vi "RTS Read System CFG.vi"(8 "Error In":errorcluster, 11 "Room CFG File Path":path) -> (0 "error out":errorcluster, 2 "Output Configuration":T1, 3 "Search File Path":path)   [LabVIEW 2020]
uses:
  Type Definitions/RTS Configuration Setup.ctl
  Type Definitions/RTS Wago Config.ctl
  Type Definitions/RTS APLUS Config.ctl
  Type Definitions/RTS Yokogawa MX Config.ctl
  Type Definitions/RTS Replay Server Control.ctl
  Type Definitions/RTS Server Configuration.ctl
  Type Definitions/RTS Station Settions TCP Comms.ctl
  Type Definitions/RTS Chamber Save Status.ctl
  Type Definitions/RTS Test Pattern.ctl
  <vilib>/Utility/file.llb/Read Delimited Spreadsheet (string).vi
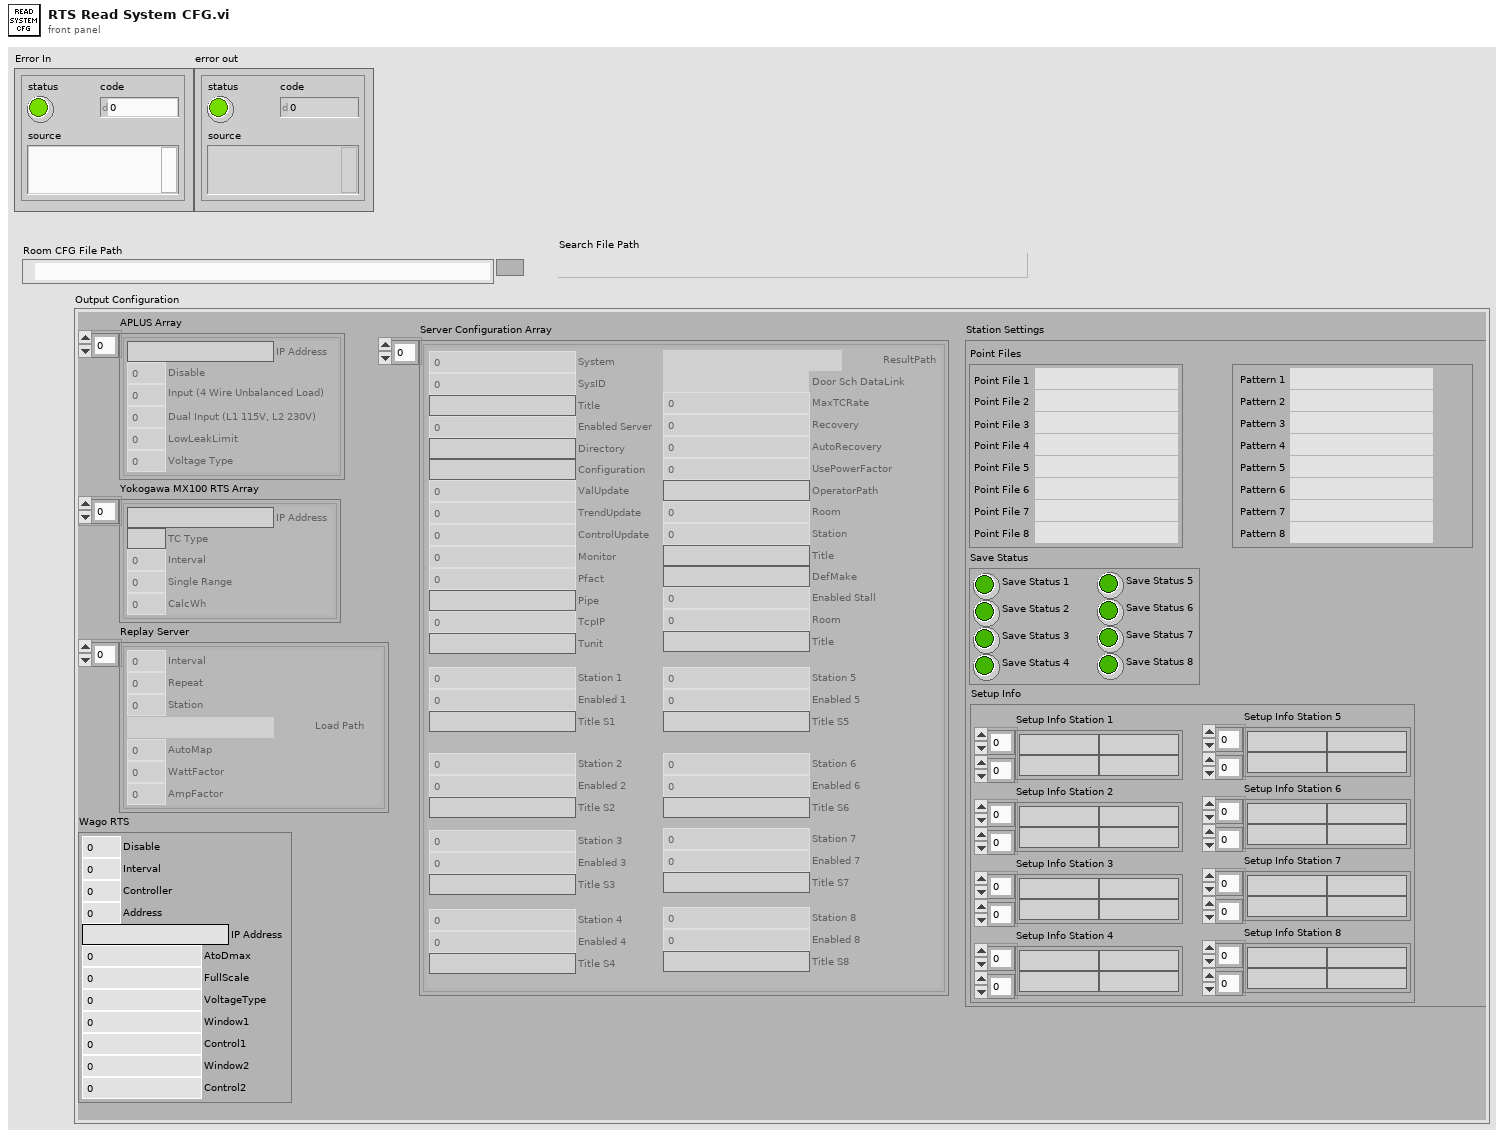
[diagram p1: front panel]
types:
  T1 = typedef "RTS Configuration Setup.ctl" = cluster{"Wago RTS":T2, "APLUS Array":T3[], "Yokogawa MX100 RTS Array":T4[], "Replay Server":T5[], "Server Configuration Array":T6[], "Station Settings":T7}
  T2 = typedef "RTS Wago Config.ctl" = cluster{"Disable":u16, "Interval":u16, "Controller":u16, "Address":u16, "IP Address":string, "AtoDmax":u16, "FullScale":u16, "VoltageType":u16, "Window1":u16, "Control1":u16, "Window2":u16, "Control2":u16}
  T3 = typedef "RTS APLUS Config.ctl" = cluster{"Disable":u16, "IP Address":string, "Input (4 Wire Unbalanced Load)":u16, "Dual Input (L1 115V, L2 230V)":u16, "LowLeakLimit":dbl, "Voltage Type":u16}
  T4 = typedef "RTS Yokogawa MX Config.ctl" = cluster{"IP Address":string, "TC Type":string, "Interval":u16, "Single Range":u16, "CalcWh":u16}
  T5 = typedef "RTS Replay Server Control.ctl" = cluster{"Interval":i16, "Repeat":u16, "Station":u16, "Load Path":path, "AutoMap":u16, "WattFactor":dbl, "AmpFactor":dbl}
  T6 = typedef "RTS Server Configuration.ctl" = cluster{"System":u16, "SysID":u16, "Title":string, "Enabled Server":u16, "Directory":string, "Configuration":string, "ValUpdate":u16, "TrendUpdate":u16, "ControlUpdate":u16, "Monitor":u16, "Pfact":u16, "Pipe":string, "TcpIP":u16, "Tunit":string, "ResultPath":path, "Door Sch DataLink":path, "MaxTCRate":u16, "Recovery":u16, "AutoRecovery":u16, "UsePowerFactor":u16, "OperatorPath":string, "Room":u16, "Station":u16, "Title":string, "DefMake":string, "Enabled Stall":u16, "Room":u16, "Title":string, "Station 1":u16, "Enabled 1":u16, "Station 2":u16, "Enabled 2":u16, "Station 3":u16, "Enabled 3":u16, "Station 4":u16, "Enabled 4":u16, "Station 5":u16, "Enabled 5":u16, "Station 6":u16, "Enabled 6":u16, "Station 7":u16, "Enabled 7":u16, "Station 8":u16, "Enabled 8":u16, "Title S1":string, "Title S2":string, "Title S3":string, "Title S5":string, "Title S6":string, "Title S7":string, "Title S8":string, "Title S4":string}
  T7 = typedef "RTS Station Settions TCP Comms.ctl" = cluster{"Point Files":cluster{"Point File 1":path, "Point File 2":path, "Point File 3":path, "Point File 4":path, "Point File 5":path, "Point File 6":path, "Point File 7":path, "Point File 8":path}, "Save Status":T8, "Setup Info":cluster{"Setup Info Station 1":string[][], "Setup Info Station 2":string[][], "Setup Info Station 3":string[][], "Setup Info Station 4":string[][], "Setup Info Station 5":string[][], "Setup Info Station 6":string[][], "Setup Info Station 7":string[][], "Setup Info Station 8":string[][]}, "Chamber Test Pattern":T9}
  T8 = typedef "RTS Chamber Save Status.ctl" = cluster{"Save Status 1":bool, "Save Status 2":bool, "Save Status 3":bool, "Save Status 4":bool, "Save Status 5":bool, "Save Status 6":bool, "Save Status 7":bool, "Save Status 8":bool}
  T9 = typedef "RTS Test Pattern.ctl" = cluster{" Pattern 1":path, "Pattern 2":path, "Pattern 3":path, "Pattern 4":path, "Pattern 5":path, "Pattern 6":path, "Pattern 7":path, "Pattern 8":path}
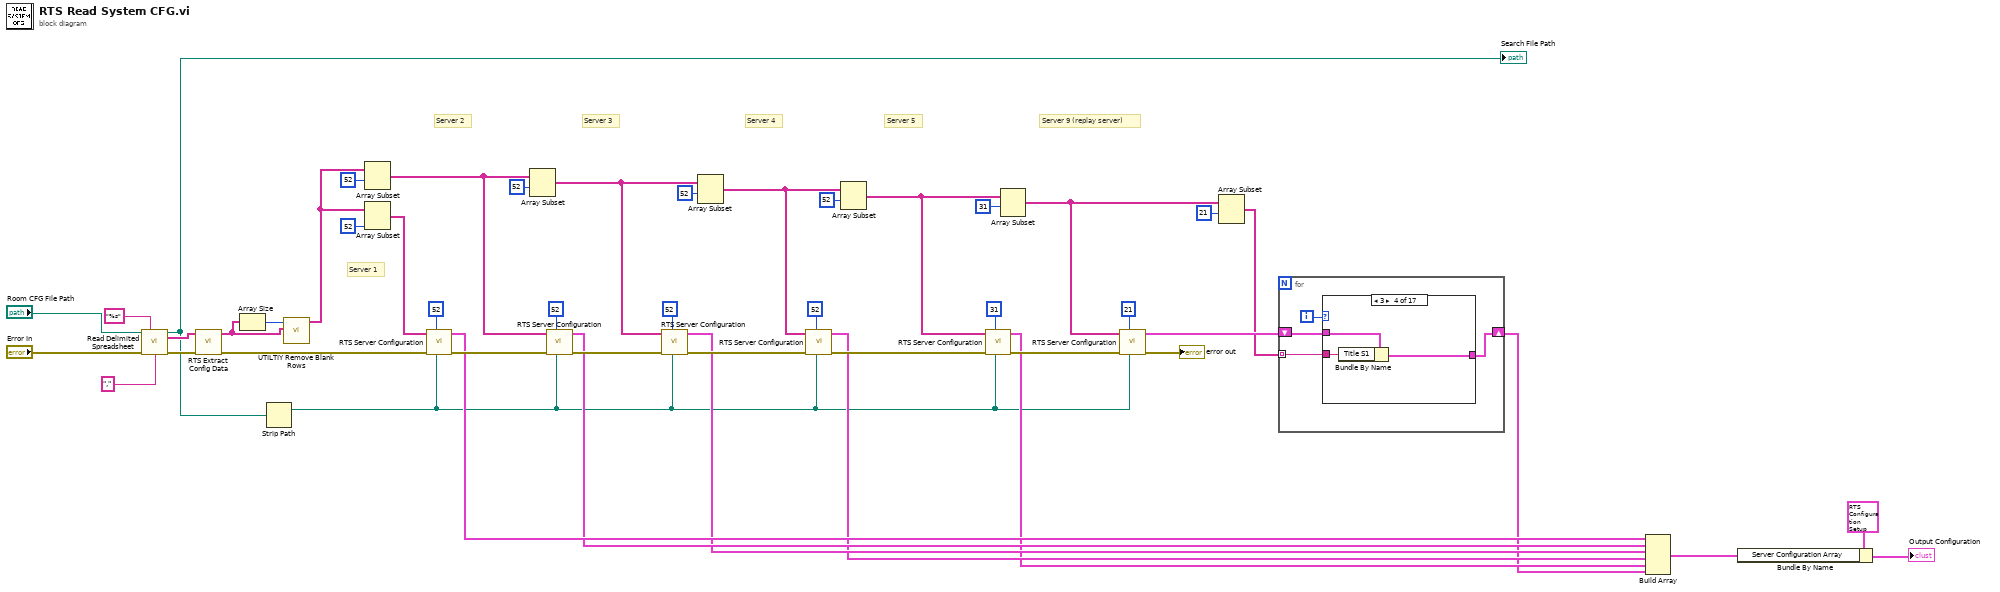
[diagram p0: block diagram]
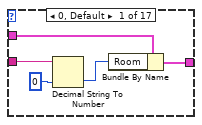
[diagram p2: hidden frame]
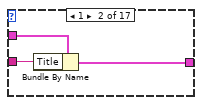
[diagram p3: hidden frame]
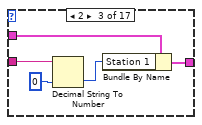
[diagram p4: hidden frame]
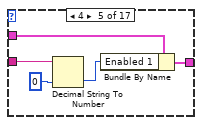
[diagram p5: hidden frame]
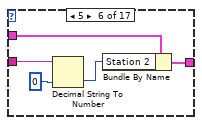
[diagram p6: hidden frame]
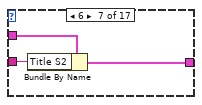
[diagram p7: hidden frame]
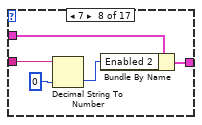
[diagram p8: hidden frame]
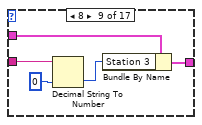
[diagram p9: hidden frame]
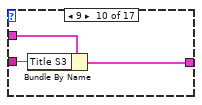
[diagram p10: hidden frame]
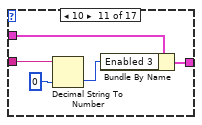
[diagram p11: hidden frame]
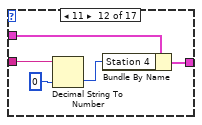
[diagram p12: hidden frame]
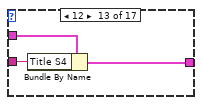
[diagram p13: hidden frame]
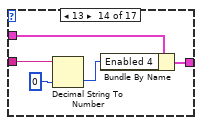
[diagram p14: hidden frame]
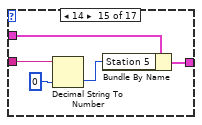
[diagram p15: hidden frame]
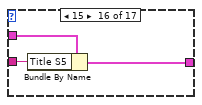
[diagram p16: hidden frame]
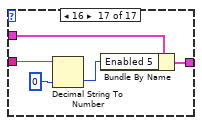
[diagram p17: hidden frame]
diagram:
  # "Server 9 (replay server)"
  # "Server 5"
  # "Server 4"
  # "Server 3"
  # "Server 2"
  # "Server 1"
  n1 = call-poly <vilib>:"Read Delimited Spreadsheet.vi"("file path (dialog if empty)"="Room CFG File Path", "format (%s)"="%s", "error in (no error)"="Error In", "delimiter (\\t)"="," ("delimiter (\\t)")) -> ("new file path (Not A Path if cancelled)"=w2:path, "all rows"=w44:string[][], "error out"=w30:errorcluster)  [unwired: 6 in, 3 out]
  "Search File Path" <- w2
  n2 = call "RTS Extract Config Data.vi"("Error In"=w30, "all rows"=w44) -> ("Error Out"=w29:errorcluster, "Array"=w43:string[])  [unwired: 8 in]
  n3 = Array Size(array=w43) -> (size(s)=w42:i32)
  n4 = Strip Path(path=w2) -> (stripped path=w1:path)  [unwired: 1 out]
  n5 = call "UTILTIY Remove Blank Rows.vi"("all rows in"=w43, "Numeric"=w42) -> ("all rows out"=w40:string[])  [unwired: 9 in]
  n6 = Array Subset(array=w40, index=52) -> (w34:string[])  [unwired: 1 in]
  n7 = Array Subset(array=w40, length=52 ("index")) -> (w35:string[])  [unwired: 1 in]
  n8 = call "RTS Server Configuration.vi"("Base Path"=w1, "Index Number"=52, "Error In"=w29, "String Data"=w35) -> ("Error Out"=w28:errorcluster, "Server Configuration"=w11:T6)  [unwired: 6 in]
  n9 = Array Subset(array=w34, index=52) -> (w33:string[])  [unwired: 1 in]
  n10 = call "RTS Server Configuration.vi"("Base Path"=w1, "Index Number"=52, "Error In"=w28, "String Data"=w34) -> ("Error Out"=w27:errorcluster, "Server Configuration"=w10:T6)  [unwired: 6 in]
  n11 = call "RTS Server Configuration.vi"("Base Path"=w1, "Index Number"=52, "Error In"=w27, "String Data"=w33) -> ("Error Out"=w26:errorcluster, "Server Configuration"=w9:T6)  [unwired: 6 in]
  n12 = Array Subset(array=w33, index=52) -> (w32:string[])  [unwired: 1 in]
  n13 = call "RTS Server Configuration.vi"("Base Path"=w1, "Index Number"=52, "Error In"=w26, "String Data"=w32) -> ("Error Out"=w25:errorcluster, "Server Configuration"=w8:T6)  [unwired: 6 in]
  n14 = Array Subset(array=w32, index=52) -> (w31:string[])  [unwired: 1 in]
  n15 = call "RTS Server Configuration.vi"("Base Path"=w1, "Index Number"=31, "Error In"=w25, "String Data"=w31) -> ("Error Out"=w17:errorcluster, "Server Configuration"=w7:T6)  [unwired: 6 in]
  n16 = Array Subset(array=w31, index=31) -> (w14:string[])  [unwired: 1 in]
  n17 = call "RTS Server Configuration.vi"("Base Path"=w1, "Index Number"=21, "Error In"=w17, "String Data"=w14) -> ("Error Out"=→"error out":errorcluster, "Server Configuration"=w15:T6)  [unwired: 6 in]
  n18 = Array Subset(array=w14, index=21) -> (w12:string[])  [unwired: 1 in]
  n19 = for {
    tunnel: w12 -> [w49] mode=indexing
    shift-right: [w50] -> w6
    shift-left: w15 -> [w51]
    i -> [w52]
    n20 = case shown="3" w52 {
      tunnel: w51 -> [w57 w60 w65 w68 w73 w78 w81 w86 w91 w94 w99 w104 w107 w112 w117 w120 w125]
      tunnel: [w56 w59 w64 w67 w72 w77 w80 w85 w90 w93 w98 w103 w106 w111 w116 w119 w124] -> w50
      tunnel: w49 -> [w55 w58 w63 w66 w71 w76 w79 w84 w89 w92 w97 w102 w105 w110 w115 w118 w123]
      frame 0, Default {
        n21 = Decimal String To Number(string=w55, default (0L)=u16 0 ("default (0 I32)")) -> (number=w54:u16)  [unwired: 1 in, 1 out]
        n22 = Bundle By Name(cluster=w57, "Room"=w54) -> (w56:T6)
      }
      frame 1 {
        n23 = Bundle By Name(cluster=w60, "Title"=w58) -> (w59:T6)
      }
      frame 2 {
        n24 = Decimal String To Number(string=w63, default (0L)=u16 0 ("default (0 I32)")) -> (number=w62:u16)  [unwired: 1 in, 1 out]
        n25 = Bundle By Name(cluster=w65, "Station 1"=w62) -> (w64:T6)
      }
      frame 3 {
        n26 = Bundle By Name(cluster=w68, "Title S1"=w66) -> (w67:T6)
      }
      frame 4 {
        n27 = Decimal String To Number(string=w71, default (0L)=u16 0 ("default (0 I32)")) -> (number=w70:u16)  [unwired: 1 in, 1 out]
        n28 = Bundle By Name(cluster=w73, "Enabled 1"=w70) -> (w72:T6)
      }
      frame 5 {
        n29 = Decimal String To Number(string=w76, default (0L)=u16 0 ("default (0 I32)")) -> (number=w75:u16)  [unwired: 1 in, 1 out]
        n30 = Bundle By Name(cluster=w78, "Station 2"=w75) -> (w77:T6)
      }
      frame 6 {
        n31 = Bundle By Name(cluster=w81, "Title S2"=w79) -> (w80:T6)
      }
      frame 7 {
        n32 = Decimal String To Number(string=w84, default (0L)=u16 0 ("default (0 I32)")) -> (number=w83:u16)  [unwired: 1 in, 1 out]
        n33 = Bundle By Name(cluster=w86, "Enabled 2"=w83) -> (w85:T6)
      }
      frame 8 {
        n34 = Decimal String To Number(string=w89, default (0L)=u16 0 ("default (0 I32)")) -> (number=w88:u16)  [unwired: 1 in, 1 out]
        n35 = Bundle By Name(cluster=w91, "Station 3"=w88) -> (w90:T6)
      }
      frame 9 {
        n36 = Bundle By Name(cluster=w94, "Title S3"=w92) -> (w93:T6)
      }
      frame 10 {
        n37 = Decimal String To Number(string=w97, default (0L)=u16 0 ("default (0 I32)")) -> (number=w96:u16)  [unwired: 1 in, 1 out]
        n38 = Bundle By Name(cluster=w99, "Enabled 3"=w96) -> (w98:T6)
      }
      frame 11 {
        n39 = Decimal String To Number(string=w102, default (0L)=u16 0 ("default (0 I32)")) -> (number=w101:u16)  [unwired: 1 in, 1 out]
        n40 = Bundle By Name(cluster=w104, "Station 4"=w101) -> (w103:T6)
      }
      frame 12 {
        n41 = Bundle By Name(cluster=w107, "Title S4"=w105) -> (w106:T6)
      }
      frame 13 {
        n42 = Decimal String To Number(string=w110, default (0L)=u16 0 ("default (0 I32)")) -> (number=w109:u16)  [unwired: 1 in, 1 out]
        n43 = Bundle By Name(cluster=w112, "Enabled 4"=w109) -> (w111:T6)
      }
      frame 14 {
        n44 = Decimal String To Number(string=w115, default (0L)=u16 0 ("default (0 I32)")) -> (number=w114:u16)  [unwired: 1 in, 1 out]
        n45 = Bundle By Name(cluster=w117, "Station 5"=w114) -> (w116:T6)
      }
      frame 15 {
        n46 = Bundle By Name(cluster=w120, "Title S5"=w118) -> (w119:T6)
      }
      frame 16 {
        n47 = Decimal String To Number(string=w123, default (0L)=u16 0 ("default (0 I32)")) -> (number=w122:u16)  [unwired: 1 in, 1 out]
        n48 = Bundle By Name(cluster=w125, "Enabled 5"=w122) -> (w124:T6)
      }
    }
  }
  n49 = Build Array(w11, w10, w9, w8, w7, w6) -> (w4:T6[])
  n50 = Bundle By Name(cluster=T1 {"Wago RTS"={"Disable"=0, "Interval"=0, "Controller"=0, "Address"=0, "IP Address"="", "AtoDmax"=0, "FullScale"=0, "VoltageType"=0, "Window1"=0, "Control1"=0, "Window2"=0, "Control2"=0}, "APLUS Array"=[], "Yokogawa MX100 RTS Array"=[], "Replay Server"=[], "Server Configuration Array"=[], "Station Settings"={"Point Files"={"Point File 1"=path "", "Point File 2"=path "", "Point File 3"=path "", "Point File 4"=path "", "Point File 5"=path "", "Point File 6"=path "", "Point File 7"=path "", "Point File 8"=path ""}, "Save Status"={"Save Status 1"=FALSE, "Save Status 2"=FALSE, "Save Status 3"=FALSE, "Save Status 4"=FALSE, "Save Status 5"=FALSE, "Save Status 6"=FALSE, "Save Status 7"=FALSE, "Save Status 8"=FALSE}, "Setup Info"={"Setup Info Station 1"=[], "Setup Info Station 2"=[], "Setup Info Station 3"=[], "Setup Info Station 4"=[], "Setup Info Station 5"=[], "Setup Info Station 6"=[], "Setup Info Station 7"=[], "Setup Info Station 8"=[]}, "Chamber Test Pattern"={" Pattern 1"=path "", "Pattern 2"=path "", "Pattern 3"=path "", "Pattern 4"=path "", "Pattern 5"=path "", "Pattern 6"=path "", "Pattern 7"=path "", "Pattern 8"=path ""}}} ("RTS Config Setup"), "Server Configuration Array"=w4) -> (→"Output Configuration":T1)
